vi "processUseControlBodyOnlyFlag_end.vi"(4 "captionVisibilityList":bool[](array[boolean]), 6 "LabelVisibilityList":bool[](array[boolean]), 7 "useControlBodyOnly":bool, 8 "error in (no error)":errorcluster, 11 "refList":refnum<vi>[](array[refnum])) -> (0 "error out":errorcluster, 3 "refList(dup)":refnum<vi>[](array[refnum]))   [LabVIEW 2023, in "TLC_Geometry.lvlib"]
uses:
  TLC_Geometry.lvlib
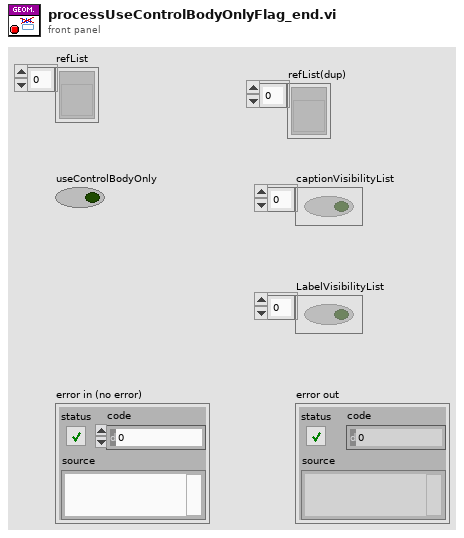
[diagram p1: front panel]
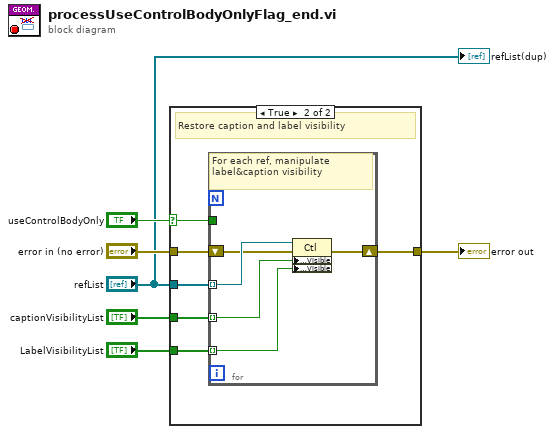
[diagram p0: block diagram]
diagram:
  n1 = case shown="True" "useControlBodyOnly" {
    selector: "useControlBodyOnly" -> [_ w11]
    tunnel: [w7 w13] -> w1
    tunnel: "error in (no error)" -> [w7 w12]
    tunnel: "LabelVisibilityList" -> [_ w10]
    tunnel: "refList" -> [_ w9]
    tunnel: "captionVisibilityList" -> [_ w8]
    frame False {
      # "Nothing to do"
    }
    frame True {
      # "Restore caption and label visibility"
      n2 = for {
        tunnel: w9 -> [w18] mode=indexing
        shift-right: [w16] -> w13
        shift-left: w12 -> [w17]
        tunnel: w11 -> [_]
        tunnel: w8 -> [w15] mode=indexing
        tunnel: w10 -> [w14] mode=indexing
        # "For each ref, manipulate label&caption visibility"
        n3 = property class="Ctl"(reference=w18, error in=w17, "Caption.Visible"=w15, "Label.Visible"=w14) -> (error out=w16:errorcluster)  [unwired: 1 out]
      }
    }
  }
  "error out" <- w1
  "refList(dup)" <- "refList"
